vi "Create.vi"(8 "error in (no error)":errorcluster) -> (0 "error out":errorcluster, 3 "Repeat Message Control out":refnum<class "Repeat Message Control.lvclass">)   [LabVIEW 2020, in "Volatus.lvlib" / "Repeat Message Control.lvclass"]
uses:
  Repeat Message Control.lvclass
  Repeat Message Control.lvclass/Repeat Message Control.ctl
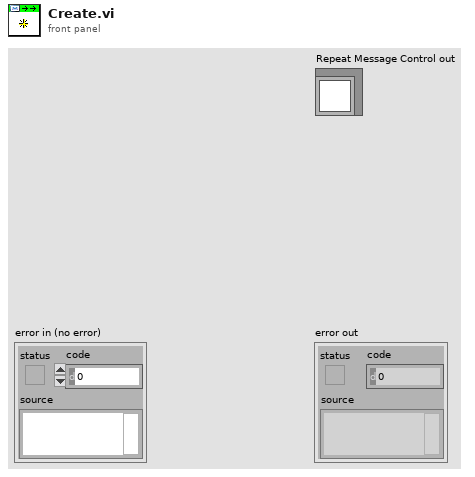
[diagram p1: front panel]
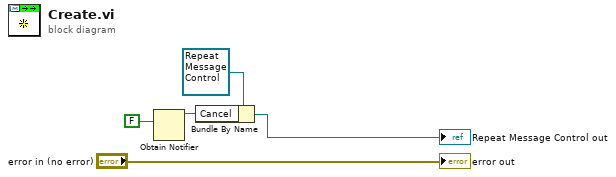
[diagram p0: block diagram]
diagram:
  n1 = Obtain Notifier(notification data type=FALSE) -> (notifier out=w1:refnum<notifier>)  [unwired: 3 in, 2 out]
  n2 = Bundle By Name(cluster=refnum<class "Repeat Message Control.lvclass"> refnum ("Repeat Message Control in"), "Cancel"=w1) -> (→"Repeat Message Control out":refnum<class "Repeat Message Control.lvclass">)
  "error out" <- "error in (no error)"
